vi "Servo MSMT LTE Configure LTE Measurements.vi"(8 "error in (no error)":errorcluster, 10 "Step In":refnum<k7>, 11 "Servo MSMT in":refnum<class "Servo MSMT.lvclass">) -> (0 "error out":errorcluster, 2 "Step Out":refnum<k7>, 3 "Servo MSMT out":refnum<class "Servo MSMT.lvclass">)   [LabVIEW 2018, in "Servo MSMT.lvlib" / "Servo MSMT.lvclass"]
uses:
  Servo MSMT.lvclass
  Servo MSMT.lvclass/Servo MSMT.ctl
  Protected Methods/Read Servo Measurements.vi
  Plugins/TestStand API Tools (TSAT).lvlibp/Step Actions/TSAT Step Actions.lvlib
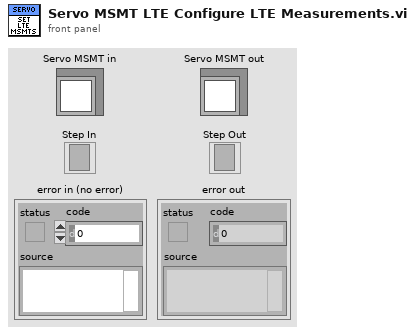
[diagram p1: front panel]
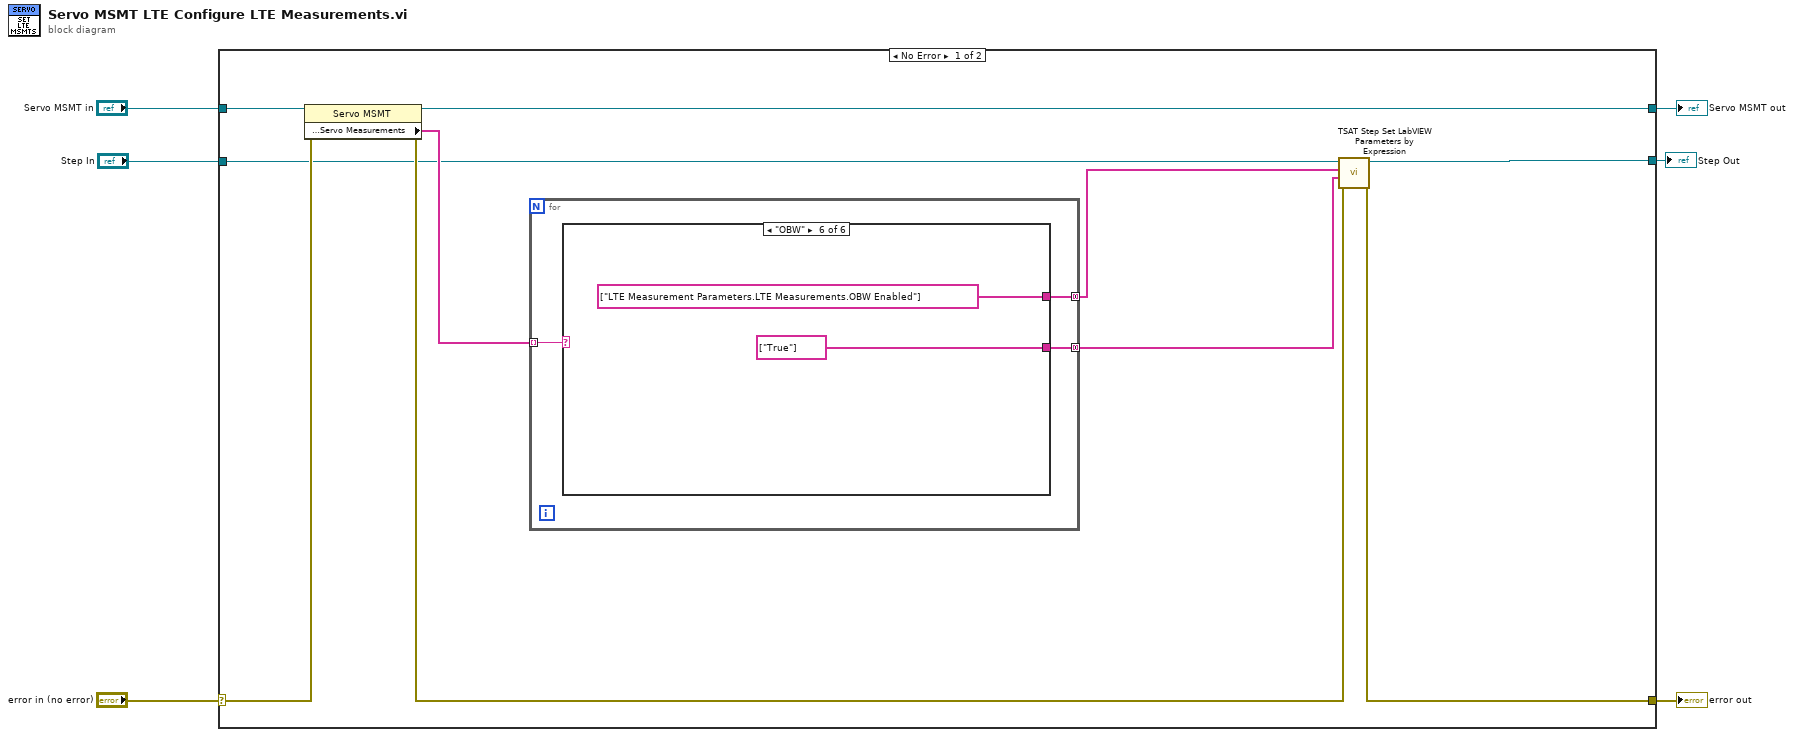
[diagram p0: block diagram]
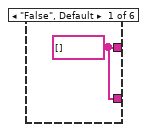
[diagram p2: hidden frame]
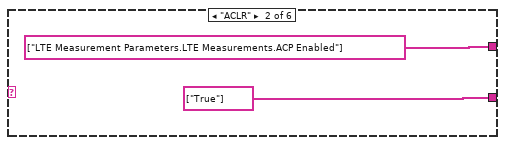
[diagram p3: hidden frame]
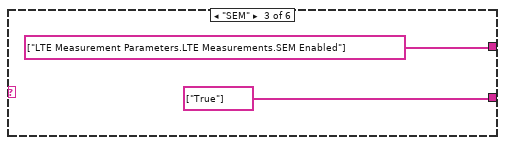
[diagram p4: hidden frame]
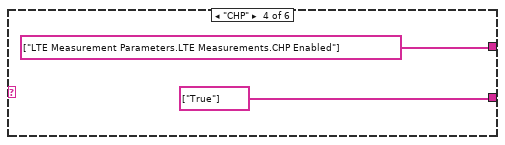
[diagram p5: hidden frame]
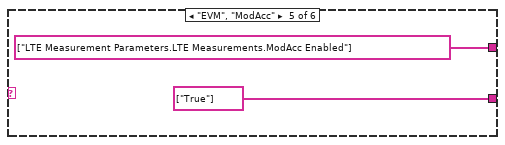
[diagram p6: hidden frame]
diagram:
  n1 = case shown="No Error" "error in (no error)" {
    selector: "error in (no error)" -> [w15 w33]
    tunnel: [w12 w33] -> w5
    tunnel: [w9 w32] -> w3
    tunnel: "Servo MSMT in" -> [w16 w32]
    tunnel: "Step In" -> [w11 w31]
    tunnel: [w10 w31] -> w1
    frame No Error {
      n2 = property class="Servo MSMT"(reference=w16, error in=w15) -> (reference out=w9:refnum<class "Servo MSMT.lvclass">, error out=w13:errorcluster, "Protected Methods:Servo Measurements"=w14:string[])
      n3 = for {
        tunnel: w14 -> [w19] mode=indexing
        tunnel: [w18] -> w8 mode=concatenating
        tunnel: [w17] -> w7 mode=concatenating
        n4 = case shown="\"OBW\"" w19 {
          tunnel: [w20 string[] ["LTE Measurement Parameters.LTE Measurements.ACP Enabled"] string[] ["LTE Measurement Parameters.LTE Measurements.SEM Enabled"] string[] ["LTE Measurement Parameters.LTE Measurements.CHP Enabled"] string[] ["LTE Measurement Parameters.LTE Measurements.ModAcc Enabled"] string[] ["LTE Measurement Parameters.LTE Measurements.OBW Enabled"]] -> w18
          tunnel: [w20 string[] ["True"] string[] ["True"] string[] ["True"] string[] ["True"] string[] ["True"]] -> w17
          frame "False", Default {
            w20 = string[] []
          }
          frame "ACLR" {
          }
          frame "SEM" {
          }
          frame "CHP" {
          }
          frame "EVM", "ModAcc" {
          }
          frame "OBW" {
          }
        }
      }
      n5 = call "TSAT Step Set LabVIEW Parameters by Expression.vi"("Error In"=w13, "Value Expressions"=w7, "Parameters to Set"=w8, "Step In"=w11) -> ("Error Out"=w12:errorcluster, "Step Out"=w10:refnum<k7>)  [unwired: 6 in]
    }
    frame Error {
    }
  }
  "error out" <- w5
  "Servo MSMT out" <- w3
  "Step Out" <- w1
